vi "Update PID.vi"(8 "error in (no error)":errorcluster, 10 "ctl":cluster{"p":dbl, "i":dbl, "d":dbl}, 11 "TEC in":refnum<class "TEC.lvclass">) -> (0 "error out":errorcluster, 3 "TEC out":refnum<class "TEC.lvclass">)   [LabVIEW 2014, in "Generic TEC.lvlib" / "TEC.lvclass"]
uses:
  TEC.lvclass
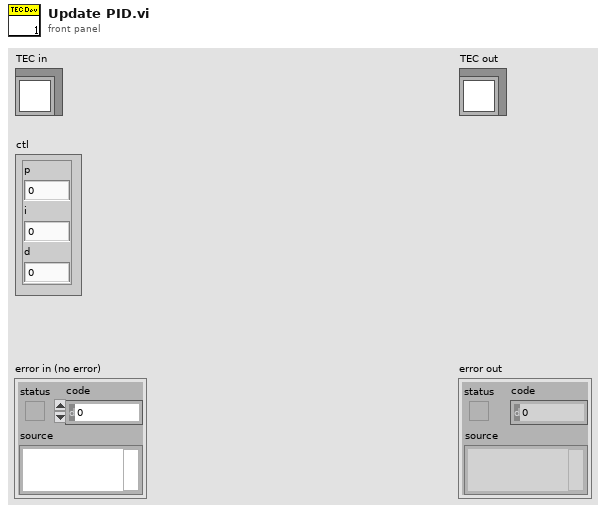
[diagram p1: front panel]
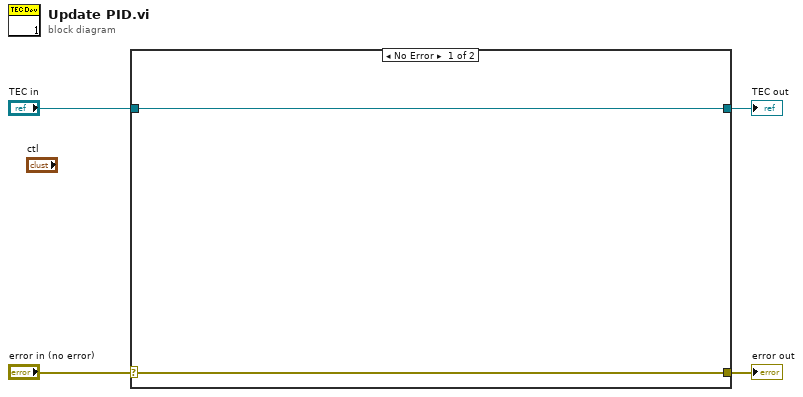
[diagram p0: block diagram]
diagram:
  n1 = case shown="No Error" "error in (no error)" {
    selector: "error in (no error)" -> [w5 w8]
    tunnel: [w5 w8] -> w3
    tunnel: [w6 w7] -> w1
    tunnel: "TEC in" -> [w6 w7]
    frame No Error {
    }
    frame Error {
    }
  }
  "error out" <- w3
  "TEC out" <- w1
